vi "Execute.RunStimulus.vi"(8 "error in (no error)":errorcluster, 11 "State Variables":T1={"NIVS.BaseLogPath"=path "", "NIVS.SystemDefinitionFile"=path "", "NIVS.Events"={"SequenceEvent"=refnum, "SystemChangeEvent"=refnum, "WorkspaceEvent"=refnum}, "NIVS.SequenceState"=enum."Idle", "NIVS.GatewayIPAddress"="", "NIVS.DataLogSpecRef"=refnum, "NIVS.DataLogManagerRef"=refnum, "NIVS.LogSessionGUID"="", "NIVS.WorkspaceManager"=refnum, "NIVS.Deployed"=FALSE, "NIVS.ProfileRef"=refnum, "NIVS.ProfileCallback"=refnum, "NIVS.SystemStateRefs"={"CustDatRef"=refnum, "EvtRef"=refnum}, "UI.Abort"=refnum, "UI.Pause"=refnum, "UI.EnableLogging"=refnum, "UI.Start"=refnum, "UI.LogChannels"=refnum, "UI.StartIteration"=refnum, "UI.StartStep"=refnum, "UI.Sequence"=refnum, "UI.PreviewMode"=refnum, "UI.Graph"=refnum, "UI.BaseFileName"=refnum, "UI.Profiles"=refnum, "UI.CurrentStep"=refnum, "UI.CurrentIteration"=refnum, "UI.TotalIterations"=refnum, "Sequence.AbortChannel"="", "Sequence.StepInfoChannel"="", "Sequence.Iterations"=0, "Sequence.IterationInfoChannel"="", "Sequence.#ofColumns"=0, "Events.State"=refnum, "Events.Test Result"=refnum, "Events.Progress"=refnum, "INI.Settings"={"Build Location"=path "C:/Simple Sequence Editor/SequenceRepo", "LoggingLocation"=path ""}}) -> (0 "error out":errorcluster, 3 "State Variables":T1={"NIVS.BaseLogPath"=path "", "NIVS.SystemDefinitionFile"=path "", "NIVS.Events"={"SequenceEvent"=refnum, "SystemChangeEvent"=refnum, "WorkspaceEvent"=refnum}, "NIVS.SequenceState"=enum."Idle", "NIVS.GatewayIPAddress"="", "NIVS.DataLogSpecRef"=refnum, "NIVS.DataLogManagerRef"=refnum, "NIVS.LogSessionGUID"="", "NIVS.WorkspaceManager"=refnum, "NIVS.Deployed"=FALSE, "NIVS.ProfileRef"=refnum, "NIVS.ProfileCallback"=refnum, "NIVS.SystemStateRefs"={"CustDatRef"=refnum, "EvtRef"=refnum}, "UI.Abort"=refnum, "UI.Pause"=refnum, "UI.EnableLogging"=refnum, "UI.Start"=refnum, "UI.LogChannels"=refnum, "UI.StartIteration"=refnum, "UI.StartStep"=refnum, "UI.Sequence"=refnum, "UI.PreviewMode"=refnum, "UI.Graph"=refnum, "UI.BaseFileName"=refnum, "UI.Profiles"=refnum, "UI.CurrentStep"=refnum, "UI.CurrentIteration"=refnum, "UI.TotalIterations"=refnum, "Sequence.AbortChannel"="", "Sequence.StepInfoChannel"="", "Sequence.Iterations"=0, "Sequence.IterationInfoChannel"="", "Sequence.#ofColumns"=0, "Events.State"=refnum, "Events.Test Result"=refnum, "Events.Progress"=refnum, "INI.Settings"={"Build Location"=path "C:/Simple Sequence Editor/SequenceRepo", "LoggingLocation"=path ""}})   [LabVIEW 2013, in "Simple Sequence Tools - Execution.lvlib"]
uses:
  Simple Sequence Tools - Execution.lvlib
  Types/Main.StateVariables.ctl
  Types/Execute.UserEventRefs.ctl
  <vilib>/NI Veristand/Execution/Workspace/SystemStateRegEventRef.ctl
  Types/Execution.SequenceState.ctl
  <vilib>/NI Veristand/Execution/DataLogging/DataLoggingSpecification Ref.ctl
  NationalInstruments.VeriStand.ClientAPI
  <vilib>/NI Veristand/Execution/DataLogging/IDataLogging Ref.ctl
  <vilib>/NI Veristand/Execution/Workspace/WorkspaceAPI.ctl
  NationalInstruments.VeriStand.RealTimeSequenceDefinitionApi
  <vilib>/NI Veristand/Execution/Workspace/SystemStateEventRef.ctl
  Shared/Types/INI.Settings
  NationalInstruments.VeriStand.DataTypes
  <vilib>/NI Veristand/Execution/DataLogging/TDMS Channel Group.ctl
  <vilib>/NI Veristand/Execution/DataLogging/TDMS Property.ctl
  <vilib>/NI Veristand/Execution/DataLogging/TDMS Channel.ctl
  <vilib>/NI Veristand/Execution/DataLogging/Time Channel Options.ctl
  <vilib>/NI Veristand/Execution/DataLogging/File Conflict Operation.ctl
  Shared/SubVIs/Main.Constants.vi
  <vilib>/NI Veristand/Execution/DataLogging/New Data Logging Specification (TDMS).vi
  <vilib>/NI Veristand/Execution/DataLogging/Set Data Logging Rate (Target Rate).vi
  <vilib>/NI Veristand/Execution/DataLogging/Set Start Trigger (Start Immediately).vi
  <vilib>/NI Veristand/Execution/Workspace/NI_VS Workspace ExecutionAPI.lvlib
  Shared/Simple Sequence Tools - Shared.lvlib
  <vilib>/NI Veristand/Execution/DataLogging/NI_VS Data Logging API.lvlib
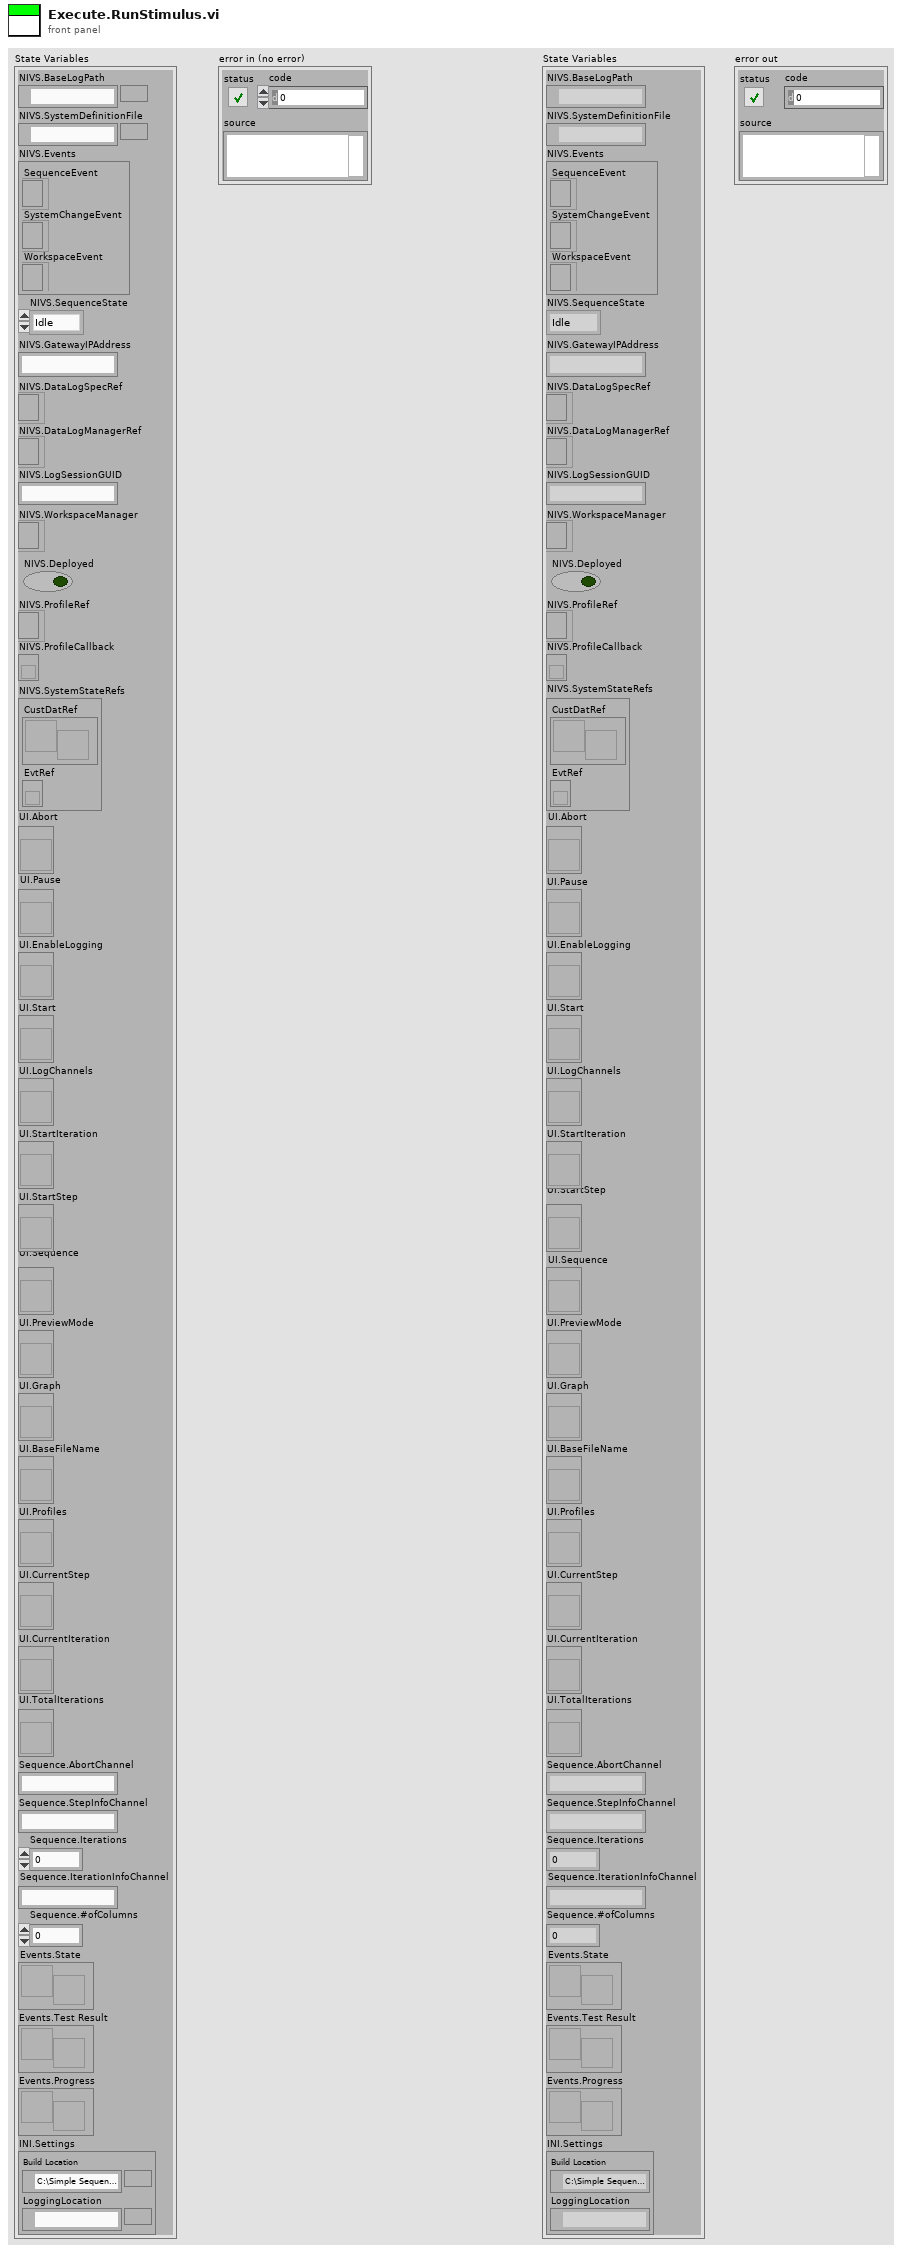
[diagram p1: front panel]
types:
  T1 = typedef "Simple Sequence Tools - Execution.lvlib/Main.StateVariables.ctl" = cluster{"NIVS.BaseLogPath":path, "NIVS.SystemDefinitionFile":path, "NIVS.Events":T2, "NIVS.SequenceState":T4, "NIVS.GatewayIPAddress":string, "NIVS.DataLogSpecRef":T5, "NIVS.DataLogManagerRef":T6, "NIVS.LogSessionGUID":string, "NIVS.WorkspaceManager":T7, "NIVS.Deployed":bool, "NIVS.ProfileRef":refnum<k24>, "NIVS.ProfileCallback":refnum<k27>, "NIVS.SystemStateRefs":T8, "UI.Abort":refnum<vi>, "UI.Pause":refnum<vi>, "UI.EnableLogging":refnum<vi>, "UI.Start":refnum<vi>, "UI.LogChannels":refnum<vi>, "UI.StartIteration":refnum<vi>, "UI.StartStep":refnum<vi>, "UI.Sequence":refnum<vi>, "UI.PreviewMode":refnum<vi>, "UI.Graph":refnum<vi>, "UI.BaseFileName":refnum<vi>, "UI.Profiles":refnum<vi>, "UI.CurrentStep":refnum<vi>, "UI.CurrentIteration":refnum<vi>, "UI.TotalIterations":refnum<vi>, "Sequence.AbortChannel":string, "Sequence.StepInfoChannel":string, "Sequence.Iterations":u32, "Sequence.IterationInfoChannel":string, "Sequence.#ofColumns":i32, "Events.State":refnum<user-event>, "Events.Test Result":refnum<user-event>, "Events.Progress":refnum<user-event>, "INI.Settings":T9}
  T2 = typedef "Simple Sequence Tools - Execution.lvlib/Execute.UserEventRefs.ctl" = cluster{"SequenceEvent":refnum<event-registration>, "SystemChangeEvent":T3, "WorkspaceEvent":refnum<event-registration>}
  T3 = typedef "NI_VS Workspace ExecutionAPI.lvlib/SystemStateRegEventRef.ctl" = refnum<event-registration>
  T4 = typedef "Simple Sequence Tools - Execution.lvlib/Execution.SequenceState.ctl" = enum16{"Idle", "Initializing", "Running", "Paused", "Finalizing", "Complete"}
  T5 = typedef "NI_VS Data Logging API.lvlib/DataLoggingSpecification Ref.ctl" = refnum<k24>
  T6 = typedef "NI_VS Data Logging API.lvlib/IDataLogging Ref.ctl" = refnum<k24>
  T7 = typedef "NI_VS Workspace ExecutionAPI.lvlib/WorkspaceAPI.ctl" = refnum<k24>
  T8 = typedef "NI_VS Workspace ExecutionAPI.lvlib/SystemStateEventRef.ctl" = cluster{"CustDatRef":refnum<user-event>, "EvtRef":refnum<k27>}
  T9 = typedef "Simple Sequence Tools - Shared.lvlib/INI.Settings" = cluster{"Build Location":path, "LoggingLocation":path}
  T10 = enum16{"Channels (No System Channel)", "Aliases", "All"}
  T11 = typedef "NI_VS Data Logging API.lvlib/File Conflict Operation.ctl" = enum16{"Create Unique", "Append to Existing", "Overwrite"}
  T12 = typedef "NI_VS Data Logging API.lvlib/Time Channel Options.ctl" = enum16{"No Time Channel", "Absolute Time", "System Time", "System Time - Microseconds", "Absolute Time as Double"}
  T13 = typedef "NI_VS Data Logging API.lvlib/TDMS Channel Group.ctl" = cluster{"Group Name":string, "Group Description":string, "Group Properties":T14[], "Channels":T15[], "Time Channel Options":T12, "Time Channel Name":string}
  T14 = typedef "NI_VS Data Logging API.lvlib/TDMS Property.ctl" = cluster{"Name":string, "Value":variant}
  T15 = typedef "NI_VS Data Logging API.lvlib/TDMS Channel.ctl" = cluster{"Channel Name":string, "Channel Path":string, "Channel Description":string, "Channel Properties":T14[]}
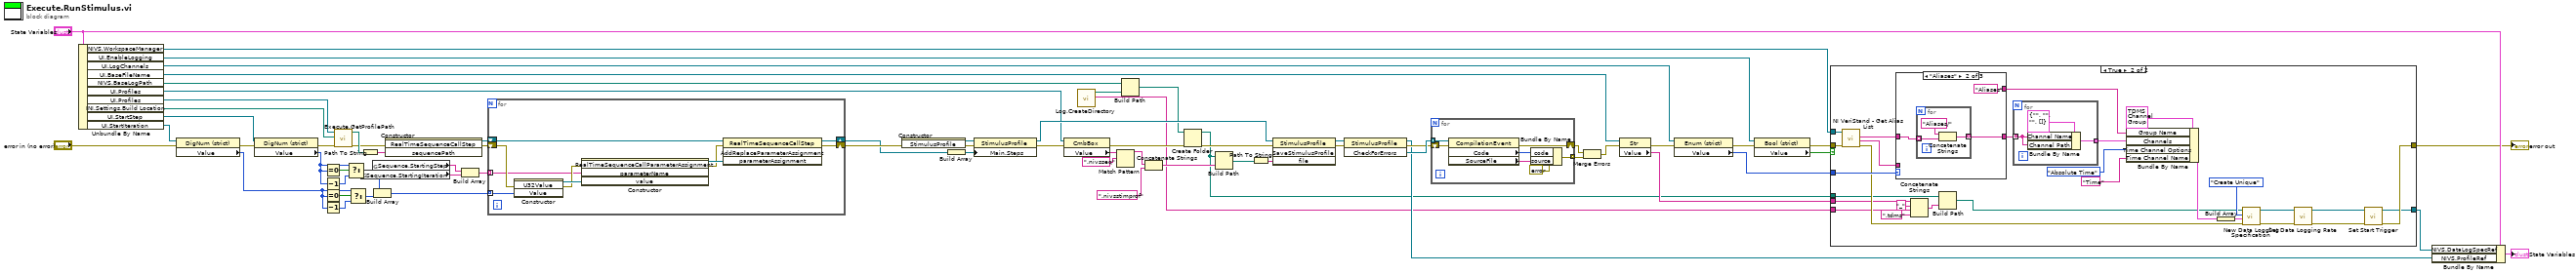
[diagram p0: block diagram]
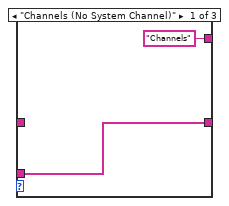
[diagram p3: hidden frame]
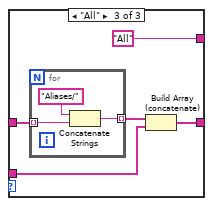
[diagram p4: hidden frame]
diagram:
  n1 = Unbundle By Name("State Variables") -> ("NIVS.WorkspaceManager"=w24:T7, "UI.EnableLogging"=w26:refnum<vi>, "UI.LogChannels"=w20:refnum<vi>, "UI.BaseFileName"=w21:refnum<vi>, "NIVS.BaseLogPath"=w15:path, "UI.Profiles"=w12:refnum<vi>, "UI.Profiles"=w61:refnum<vi>, "INI.Settings.Build Location"=w16:path, "UI.StartStep"=w42:refnum<vi>, "UI.StartIteration"=w44:refnum<vi>)
  n2 = property class="DigNum (strict)"(reference=w44, error in="error in (no error)") -> (error out=w43:errorcluster, "Value"=w30:u32)  [unwired: 1 out]
  n3 = property class="DigNum (strict)"(reference=w42, error in=w43) -> (error out=w41:errorcluster, "Value"=w36:u32)  [unwired: 1 out]
  n4 = Equal To 0?(x=w36) -> (x = 0?=w35:bool)
  n5 = Decrement(x=w36) -> (x-1=w34:u32)
  n6 = Equal To 0?(x=w30) -> (x = 0?=w31:bool)
  n7 = Decrement(x=w30) -> (x-1=w32:u32)
  n8 = call "Execute.GetProfilePath.vi"("error in (no error)"=w41, "base path"=w16, "Profiles"=w61) -> ("error out"=w64:errorcluster, "Path"=w66:path)  [unwired: 7 in]
  n9 = Select(t=w36, s=w35, f=w34) -> (s? t:f=w33:u32)
  n10 = Select(t=w30, s=w31, f=w32) -> (s? t:f=w29:u32)
  n11 = global read "Main.Constants.vi" "Sequence.StartingIteration"() -> (w38:string)
  n12 = Path To String(path=w66) -> (string=w65:string)
  n13 = global read "Main.Constants.vi" "Sequence.StartingStep"() -> (w39:string)
  n14 = Build Array(w33, w29) -> (w40:u32[])
  n15 = constructor class="RealTimeSequenceCallStep"(error in=w64, "sequencePath"=w65) -> (reference out=w47:refnum<k24>, error out=w45:errorcluster)  [unwired: 2 in, 2 out]
  n16 = Build Array(w39, w38) -> (w37:string[])
  n17 = for {
    tunnel: w37 -> [w71] mode=indexing
    tunnel: w40 -> [w69] mode=indexing
    shift-right: [w76] -> w46
    shift-left: w47 -> [w77]
    shift-right: [w78] -> w48
    shift-left: w45 -> [w72]
    n18 = constructor class="U32Value"(error in=w72, "Value"=w69) -> (reference out=w74:refnum<k24>, error out=w73:errorcluster)  [unwired: 2 in, 2 out]
    n19 = constructor class="RealTimeSequenceCallParameterAs"(error in=w73, "parameterName"=w71, "value"=w74) -> (reference out=w75:refnum<k24>, error out=w70:errorcluster)  [unwired: 2 in, 3 out]
    n20 = invoke class="RealTimeSequenceCallStep" method="AddReplaceParameterAssignment"(reference=w77, error in=w70, "parameterAssignment"=w75) -> (reference out=w76:refnum<k24>, error out=w78:errorcluster)  [unwired: 1 in, 2 out]
  }
  n21 = constructor class="StimulusProfile"(error in=w48) -> (reference out=w63:refnum<k24>, error out=w59:errorcluster)  [unwired: 2 in, 1 out]
  n22 = Build Array(w46) -> (w60:refnum<k24>[])
  n23 = property class="StimulusProfile"(reference=w63, error in=w59, "Main.Steps"=w60) -> (reference out=w28:refnum<k24>, error out=w11:errorcluster)
  n24 = property class="CmbBox"(reference=w12, error in=w11) -> (error out=w9:errorcluster, "Value"=w3:string)  [unwired: 1 out]
  n25 = call "Log.CreateDirectory.vi"() -> ("String"=w4:string, "File Folder"=w14:path)  [unwired: 10 in]
  n26 = Match Pattern(string=w3, regular expression=".nivsseq" ("string")) -> (before substring=w2:string)  [unwired: 1 in, 3 out]
  n27 = Build Path(base path=w15, name or relative path=w14) -> (appended path=w7:path)
  n28 = Concatenate Strings(w2, ".nivsstimprof" ("string")) -> (w6:string)
  n29 = Create Folder(path (use dialog)=w7, error in=w9) -> (created path=w5:path, error out=w8:errorcluster)  [unwired: 1 in, 1 out]
  n30 = Build Path(base path=w5, name or relative path=w6) -> (appended path=w13:path)
  n31 = Path To String(path=w13) -> (string=w62:string)
  n32 = invoke class="StimulusProfile" method="SaveStimulusProfile"(reference=w28, error in=w8, "file"=w62) -> (reference out=w54:refnum<k24>, error out=w53:errorcluster)  [unwired: 1 in, 2 out]
  n33 = invoke class="StimulusProfile" method="CheckForErrors"(reference=w54, error in=w53) -> (reference out=w17:refnum<k24>, error out=w51:errorcluster, "CheckForErrors"=w52:refnum<k24>[])  [unwired: 1 in]
  n34 = for {
    tunnel: w52 -> [w85] mode=indexing
    tunnel: [w80] -> w49 mode=indexing
    shift-right: [w79] -> w50
    shift-left: w51 -> [w84]
    n35 = property class="CompilationEvent"(reference=w85, error in=w84) -> (error out=w79:errorcluster, "Code"=w82:i32, "SourceFile"=w81:string)  [unwired: 1 out]
    n36 = Bundle By Name(cluster=errorcluster {"status"=TRUE, "code"=0, "source"=""} ("error out"), "code"=w82, "source"=w81) -> (w80:errorcluster)
  }
  n37 = Merge Errors(w50, w49) -> (w19:errorcluster)
  n38 = property class="Str"(reference=w21, error in=w19) -> (error out=w56:errorcluster, "Value"=w57:string)  [unwired: 1 out]
  n39 = property class="Enum (strict)"(reference=w20, error in=w56) -> (error out=w23:errorcluster, "Value"=w55:T10)  [unwired: 1 out]
  n40 = property class="Bool (strict)"(reference=w26, error in=w23) -> (error out=w25:errorcluster, "Value"=w58:bool)  [unwired: 1 out]
  n41 = case shown="True" w58 {
    tunnel: w25 -> [w86 w114]
    tunnel: [w86 w96] -> w18
    tunnel: w57 -> [_ w92]
    tunnel: w55 -> [_ w112]
    tunnel: w24 -> [_ w113]
    tunnel: [_ w95] -> w27
    tunnel: w5 -> [_ w93]
    tunnel: w4 -> [_ w88]
    frame False {
    }
    frame True {
      n42 = call <vilib>:"NI VeriStand - Get Alias List.vi"("error in (no error)"=w114, "WorkspaceManager in"=w113) -> ("error out"=w94:errorcluster, "Channels"=w109:string[], "Aliases"=w111:string[])  [unwired: 6 in, 1 out]
      n43 = case shown="\"Aliases\"" w112 {
        tunnel: w111 -> [_ w119 w127]
        tunnel: [w116 w118 w125] -> w110
        tunnel: w109 -> [w116 _ w124]
        tunnel: ["Channels" "Aliases" "All"] -> w102
        frame "Channels (No System Channel)" {
        }
        frame "Aliases" {
          n44 = for {
            tunnel: w119 -> [w122] mode=indexing
            tunnel: [w120] -> w118 mode=indexing
            n45 = Concatenate Strings("Aliases/", w122) -> (w120:string)
          }
        }
        frame "All" {
          n46 = for {
            tunnel: w127 -> [w130] mode=indexing
            tunnel: [w128] -> w126 mode=indexing
            n47 = Concatenate Strings("Aliases/", w130) -> (w128:string)
          }
          n48 = Build Array (concatenate)(w126, w124) -> (w125:string[])
        }
      }
      n49 = Concatenate Strings(w92, "_" ("string"), w88, ".tdms" ("string")) -> (w90:string)
      n50 = Build Path(base path=w93, name or relative path=w90) -> (appended path=w87:path)
      n51 = for {
        tunnel: w110 -> [w132] mode=indexing
        tunnel: [w131] -> w105 mode=indexing
        n52 = Bundle By Name(cluster=T15 {"Channel Name"="", "Channel Path"="", "Channel Description"="", "Channel Properties"=[]} ("TDMS Channel"), "Channel Name"=w132, "Channel Path"=w132) -> (w131:T15)
      }
      n53 = Bundle By Name(cluster=T13 {"Group Name"="", "Group Description"="", "Group Properties"=[], "Channels"=[], "Time Channel Options"=enum."No Time Channel", "Time Channel Name"=""} ("TDMS Channel Group"), "Group Name"=w102, "Channels"=w105, "Time Channel Options"=Time_Channel_Options."Absolute Time", "Time Channel Name"="Time") -> (w99:T13)
      n54 = Build Array(w99) -> (w98:T13[])
      n55 = call-poly <vilib>:"New Data Logging Specification.vi"("error in (no error)"=w94, "Channel Groups"=w98, "File Conflict Operation"=File_Conflict_Operation."Create Unique", "Base Log File Path"=w87) -> ("error out"=w100:errorcluster, "Data Logging Specification Ref out"=w108:T5)  [unwired: 6 in]
      n56 = call-poly <vilib>:"Set Data Logging Rate.vi"("error in (no error)"=w100, "Data Logging Specification Ref in"=w108) -> ("error out"=w101:errorcluster, "Data Logging Specification Ref out"=w107:T5)  [unwired: 8 in]
      n57 = call-poly <vilib>:"Set Start Trigger.vi"("error in (no error)"=w101, "Data Logging Specification Ref in"=w107) -> ("error out"=w96:errorcluster, "Data Logging Specification Ref out"=w95:T5)  [unwired: 8 in]
    }
  }
  "error out" <- w18
  n58 = Bundle By Name(cluster="State Variables", "NIVS.DataLogSpecRef"=w27, "NIVS.ProfileRef"=w17) -> (→"State Variables":T1)
